vi "stake master data collection .vi"(0 "Refnum in":T1, 1 "STAKEHOLDER ID":string, 2 "Select Month":string, 5 "Shift":string, 7 "total date":string[](array[string]), 9 "Select Line":string, 11 "error in (no error)":errorcluster, 12 "Select Year":string) -> (3 "Count out":string[](array[string]), 4 "Refnum out":T1, 6 "string min":string[](array[string]), 10 "DURATION SUM OF ARRAY":dbl, 14 "COUNT OF ARRAY":dbl, 15 "error out":errorcluster)   [LabVIEW 2017]
uses:
  <vilib>/addons/database/Connection.llb/Conn ObjectReference.ctl
  <vilib>/addons/database/NI_Database_API.lvlib
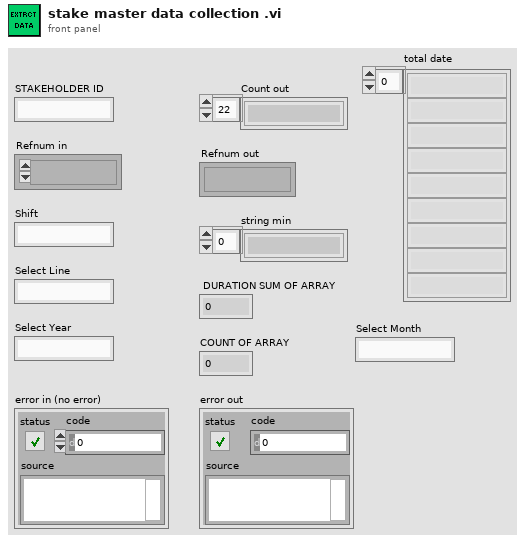
[diagram p1: front panel]
types:
  T1 = typedef "NI_Database_API.lvlib/Conn ObjectReference.ctl" = refnum<k1>
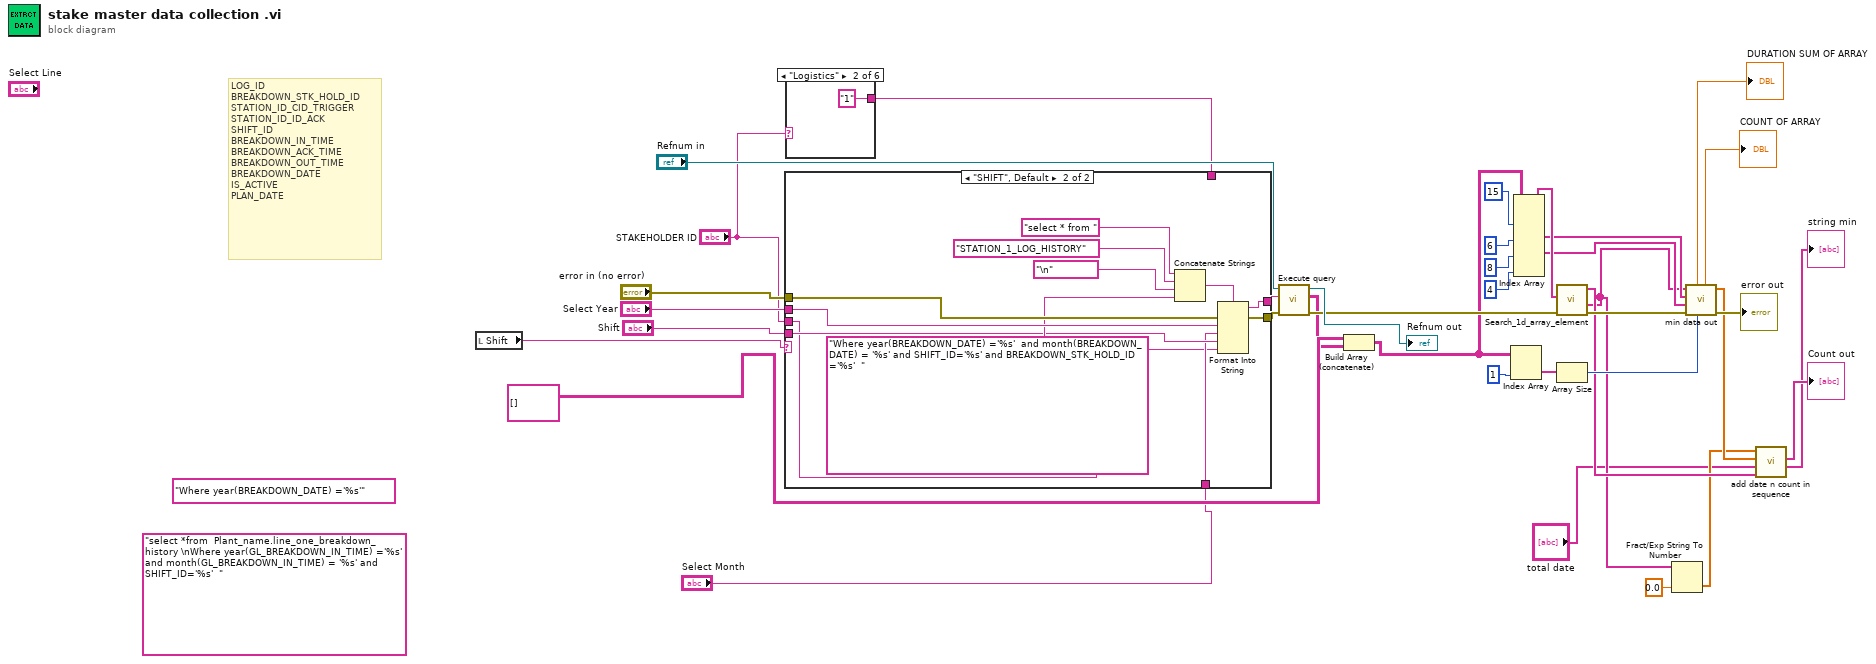
[diagram p0: block diagram]
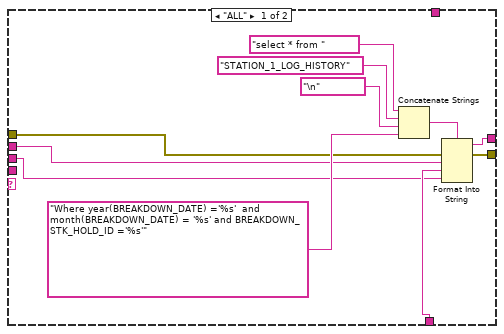
[diagram p2: hidden frame]
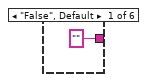
[diagram p3: hidden frame]
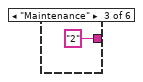
[diagram p4: hidden frame]
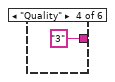
[diagram p5: hidden frame]
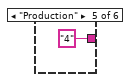
[diagram p6: hidden frame]
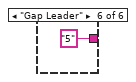
[diagram p7: hidden frame]
diagram:
  (unwired) "Where year(BREAKDOWN_DATE) ='%s'" ("condition")
  (unwired) "select *from  Plant_name.line_one_breakdown_history \nWhere year(GL_BREAKDOWN_IN_TIME) ='%s'  and month(GL_BREAKDOWN_IN_TIME) = '%s' and SHIFT_ID='%s'  " ("condition")
  # "LOG_ID\nBREAKDOWN_STK_HOLD_ID\nSTATION_ID_CID_TRIGGER\nSTATION_ID_ID_ACK\nSHIFT_ID\nBREAKDOWN_IN_TIME\nBREAKDOWN_ACK_TIME\nBREAKDOWN_OUT_TIME\nBREAKDOWN_DATE\nIS_ACTIVE\nPLAN_DATE"
  n1 = local read "Shift"() -> (w18:string)
  n2 = case shown="\"Logistics\"" "STAKEHOLDER ID" {
    tunnel: ["" "1" "2" "3" "4" "5"] -> w1
    frame "False", Default {
    }
    frame "Logistics" {
    }
    frame "Maintenance" {
    }
    frame "Quality" {
    }
    frame "Production" {
    }
    frame "Gap Leader" {
    }
  }
  n3 = case shown="\"SHIFT\", Default" w18 {
    tunnel: "error in (no error)" -> [w50 w63]
    tunnel: "Select Year" -> [w49 w62]
    tunnel: "STAKEHOLDER ID" -> [w45 w56]
    tunnel: "Shift" -> [_ w58]
    tunnel: [w48 w61] -> w3
    tunnel: [w47 w60] -> w2
    tunnel: "Select Month" -> [w46 w57]
    tunnel: w1 -> [_ _]
    frame "ALL" {
      n4 = Concatenate Strings("select * from " ("string"), "STATION_1_LOG_HISTORY" ("table"), "\n" ("string"), "Where year(BREAKDOWN_DATE) ='%s'  and month(BREAKDOWN_DATE) = '%s' and BREAKDOWN_STK_HOLD_ID ='%s'" ("condition")) -> (w54:string)
      n5 = Format Into String(format string=w54, error in=w50, w49, w46, w45) -> (resulting string=w48:string, error out=w47:errorcluster)  [unwired: 1 in]
    }
    frame "SHIFT", Default {
      n6 = Concatenate Strings("select * from " ("string"), "STATION_1_LOG_HISTORY" ("table"), "\n" ("string"), "Where year(BREAKDOWN_DATE) ='%s'  and month(BREAKDOWN_DATE) = '%s' and SHIFT_ID='%s' and BREAKDOWN_STK_HOLD_ID ='%s'  " ("condition")) -> (w66:string)
      n7 = Format Into String(format string=w66, error in=w63, w62, w57, w58, w56) -> (resulting string=w61:string, error out=w60:errorcluster)  [unwired: 1 in]
    }
  }
  n8 = call "Execute query.vi"("error in (no error)"=w2, "String"=w3, "connection reference"="Refnum in") -> ("error out"=w36:errorcluster, "Table"=w4:string[][], "connection reference 2"=→"Refnum out":T1)  [unwired: 5 in, 1 out]
  n9 = Build Array (concatenate)(string[][] [], w4) -> (w19:string[][])
  n10 = Index Array(array=w19, index (col)=1 ("disabled index (col)")) -> (element=w26:string[])  [unwired: 1 in]
  n11 = Index Array(array=w19, index (col) #1=15 ("index (row)"), index (col) #2=6 ("index (col)"), index (col) #3=8 ("index (col)"), index (col) #4=4 ("index (col)")) -> (element #1=w32:string[], element #2=w27:string[], element #3=w28:string[])  [unwired: 4 in, 1 out]
  n12 = call "Search_1d_array_element.vi"("error in (no error)"=w36, "BD Date"=w32) -> ("error out"=w31:errorcluster, "Count out"=w9:string[], "Elements Found out"=w10:string[])  [unwired: 5 in]
  n13 = Array Size(array=w26) -> (size(s)=w29:i32)
  n14 = Fract/Exp String To Number(string=w9, default (0 dbl)=0.0 ("default (0 DBL)")) -> (number=w8:dbl[])  [unwired: 2 in, 1 out]
  n15 = call "min data out.vi"("Numeric"=w29, "error in (no error)"=w31, "out time"=w28, "in time"=w27, "Count in"=w9) -> ("error out"=→"error out":errorcluster, "duration"=w11:dbl[], "COUNT OF ARRAY"=→"COUNT OF ARRAY":dbl, "DURATION SUM OF ARRAY"=→"DURATION SUM OF ARRAY":dbl)  [unwired: 2 in, 1 out]
  n16 = call "add date n count in sequence.vi"("find date"=w10, "total date"="total date", "duration"=w11, "count"=w8) -> ("DURATION"=→"string min":string[], "COUNT"=→"Count out":string[])  [unwired: 5 in, 1 out]
